vi "Sketch Plane.vi"(10 "result string in":string, 11 "Sketch Plane":T1) -> (3 "result string out":string)   [LabVIEW 2019]
uses:
  <userlib>/Onshape Feature Funcrions/_SubVI/Sketch Plane.ctl
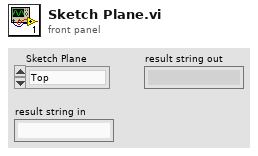
[diagram p1: front panel]
types:
  T1 = typedef "Sketch Plane.ctl" = enum16{"Top", "Front", "Right", "plane1", "plane2", "plane3"}
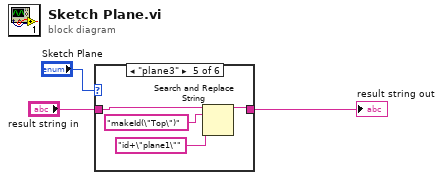
[diagram p0: block diagram]
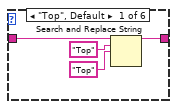
[diagram p2: hidden frame]
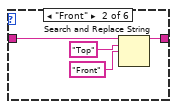
[diagram p3: hidden frame]
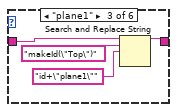
[diagram p4: hidden frame]
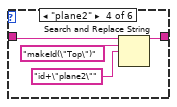
[diagram p5: hidden frame]
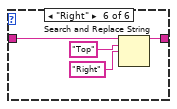
[diagram p6: hidden frame]
diagram:
  n1 = case shown="\"plane3\"" "Sketch Plane" {
    tunnel: "result string in" -> [w5 w9 w13 w17 w21 w26]
    tunnel: [w4 w8 w12 w16 w20 w24] -> w1
    frame "Top", Default {
      n2 = Search and Replace String(input string=w5, search string="Top" ("regular expression"), replace string="Top" ("regular expression")) -> (result string=w4:string)  [unwired: 5 in, 3 out]
    }
    frame "Front" {
      n3 = Search and Replace String(input string=w9, search string="Top" ("regular expression"), replace string="Front" ("regular expression")) -> (result string=w8:string)  [unwired: 5 in, 3 out]
    }
    frame "plane1" {
      n4 = Search and Replace String(input string=w13, search string="makeId(\"Top\")" ("regular expression"), replace string="id+\"plane1\"" ("regular expression")) -> (result string=w12:string)  [unwired: 5 in, 3 out]
    }
    frame "plane2" {
      n5 = Search and Replace String(input string=w17, search string="makeId(\"Top\")" ("regular expression"), replace string="id+\"plane2\"" ("regular expression")) -> (result string=w16:string)  [unwired: 5 in, 3 out]
    }
    frame "plane3" {
      n6 = Search and Replace String(input string=w21, search string="makeId(\"Top\")" ("regular expression"), replace string="id+\"plane1\"" ("regular expression")) -> (result string=w20:string)  [unwired: 5 in, 3 out]
    }
    frame "Right" {
      n7 = Search and Replace String(input string=w26, search string="Top" ("regular expression"), replace string="Right" ("regular expression")) -> (result string=w24:string)  [unwired: 5 in, 3 out]
    }
  }
  "result string out" <- w1
